vi "miss note handle.vi"(8 "song info":T2, 10 "score info":T1, 11 "next note":cluster{"1st rail":i32, "2nd rail":i32}) -> (2 "new score info":T1, 3 "new next note":cluster{"1st rail":i32, "2nd rail":i32})   [LabVIEW 2023]
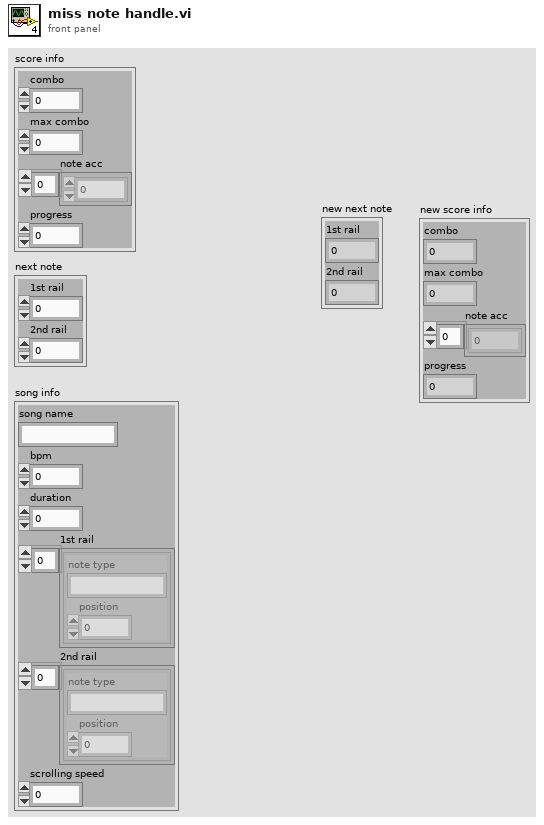
[diagram p1: front panel]
types:
  T1 = cluster{"combo":i32, "max combo":i32, "note acc":i32[], "progress":dbl}
  T2 = cluster{"song name":string, "bpm":i32, "duration":i32, "1st rail":cluster{"note type":string, "position":dbl}[], "2nd rail":cluster{"note type":string, "position":dbl}[], "scrolling speed":dbl}
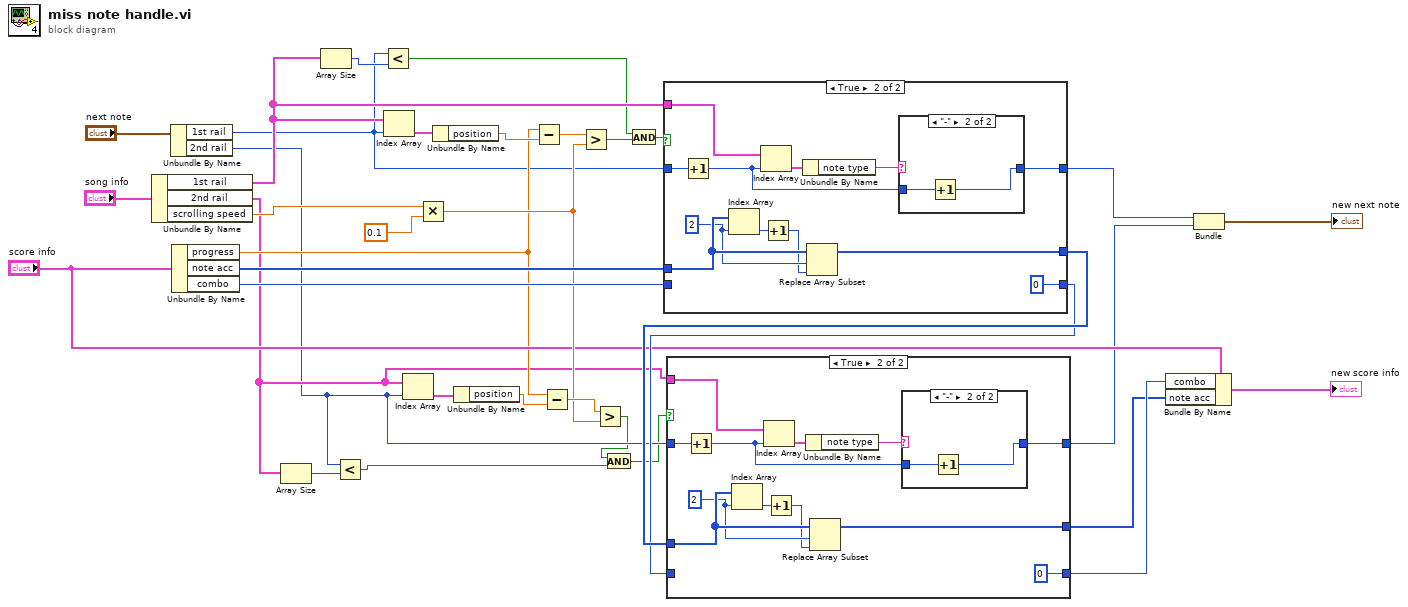
[diagram p0: block diagram]
diagram:
  n1 = Unbundle By Name("song info") -> ("1st rail"=w12:cluster{"note type":string, "position":dbl}[], "2nd rail"=w6:cluster{"note type":string, "position":dbl}[], "scrolling speed"=w31:dbl)
  n2 = Unbundle By Name("next note") -> ("1st rail"=w10:i32, "2nd rail"=w4:i32)
  n3 = Unbundle By Name("score info") -> ("progress"=w13:dbl, "note acc"=w29:i32[], "combo"=w28:i32)
  n4 = Array Size(array=w6) -> (size(s)=w5:i32)
  n5 = Array Size(array=w12) -> (size(s)=w11:i32)
  n6 = Less?(x=w4, y=w5) -> (x < y?=w1:bool)
  n7 = Less?(x=w10, y=w11) -> (x < y?=w7:bool)
  n8 = Index Array(array=w12, index=w10) -> (element=w33:cluster{"note type":string, "position":dbl})
  n9 = Index Array(array=w6, index=w4) -> (element=w27:cluster{"note type":string, "position":dbl})
  n10 = Multiply(x=w31, y=0.1) -> (x*y=w25:dbl)
  n11 = Unbundle By Name(w33) -> ("position"=w15:dbl)
  n12 = Unbundle By Name(w27) -> ("position"=w14:dbl)
  n13 = Subtract(x=w13, y=w15) -> (x-y=w32:dbl)
  n14 = Subtract(x=w13, y=w14) -> (x-y=w26:dbl)
  n15 = Greater?(x=w32, y=w25) -> (0:w8:bool)
  n16 = Greater?(x=w26, y=w25) -> (0:w2:bool)
  n17 = And(x=w2, y=w1) -> (x .and. y?=w3:bool)
  n18 = And(x=w7, y=w8) -> (x .and. y?=w9:bool)
  n19 = case shown="True" w9 {
    tunnel: w29 -> [w38 w50]
    tunnel: w10 -> [w37 w45]
    tunnel: [w38 w46] -> w24
    tunnel: [w37 w40] -> w19
    tunnel: w12 -> [_ w44]
    tunnel: w28 -> [w36 _]
    tunnel: [w36 0] -> w23
    frame False {
    }
    frame True {
      w49 = 2
      n20 = Increment(x=w45) -> (x+1=w41:i32)
      n21 = Index Array(array=w50, index=w49) -> (element=w48:i32)
      n22 = Index Array(array=w44, index=w41) -> (element=w43:cluster{"note type":string, "position":dbl})
      n23 = Increment(x=w48) -> (x+1=w47:i32)
      n24 = Unbundle By Name(w43) -> ("note type"=w42:string)
      n25 = Replace Array Subset(array=w50, new element=w47, index=w49) -> (w46:i32[])
      n26 = case shown="\"-\"" w42 {
        tunnel: w41 -> [w51 w53]
        tunnel: [w51 w52] -> w40
        frame Default {
        }
        frame "-" {
          n27 = Increment(x=w53) -> (x+1=w52:i32)
        }
      }
    }
  }
  n28 = case shown="True" w3 {
    tunnel: w24 -> [w56 w68]
    tunnel: w4 -> [w55 w63]
    tunnel: [w56 w64] -> w20
    tunnel: [w55 w58] -> w18
    tunnel: w6 -> [_ w62]
    tunnel: w23 -> [w54 _]
    tunnel: [w54 0] -> w21
    frame False {
    }
    frame True {
      w67 = 2
      n29 = Increment(x=w63) -> (x+1=w59:i32)
      n30 = Index Array(array=w68, index=w67) -> (element=w66:i32)
      n31 = Index Array(array=w62, index=w59) -> (element=w61:cluster{"note type":string, "position":dbl})
      n32 = Increment(x=w66) -> (x+1=w65:i32)
      n33 = Unbundle By Name(w61) -> ("note type"=w60:string)
      n34 = Replace Array Subset(array=w68, new element=w65, index=w67) -> (w64:i32[])
      n35 = case shown="\"-\"" w60 {
        tunnel: w59 -> [w69 w71]
        tunnel: [w69 w70] -> w58
        frame Default {
        }
        frame "-" {
          n36 = Increment(x=w71) -> (x+1=w70:i32)
        }
      }
    }
  }
  n37 = Bundle By Name(cluster="score info", "combo"=w21, "note acc"=w20) -> (→"new score info":T1)
  n38 = Bundle("1st rail"=w19, "2nd rail"=w18) -> (→"new next note":cluster{"1st rail":i32, "2nd rail":i32})  [unwired: 1 in]
